vi "F Dwf Analog Out Node Frequency Info.vi"(6 "phzMax":dbl, 7 "phzMin":dbl, 8 "error in (no error)":errorcluster, 9 "node":i32, 10 "idxChannel":i32, 11 "hdwf":i32) -> (0 "error out":errorcluster, 3 "function return":i32, 4 "phzMax out":dbl, 5 "phzMin out":dbl)   [LabVIEW 2024, in "Olasdwf.lvlib"]
doc: "DWFAPI int FDwfAnalogOutNodeFrequencyInfo(HDWF hdwf, int idxChannel, AnalogOutNode node, double *phzMin, double *phzMax);"
uses:
  Olasdwf.lvlib
  Windows/System32/dwf.dll
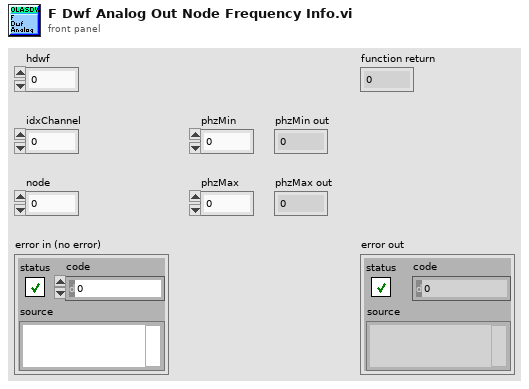
[diagram p1: front panel]
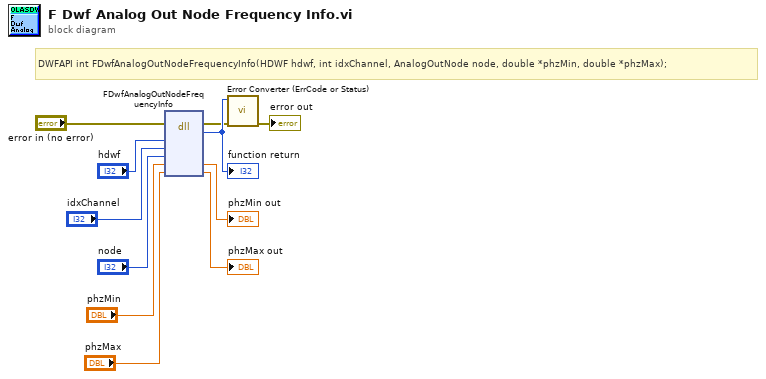
[diagram p0: block diagram]
diagram:
  # "DWFAPI int FDwfAnalogOutNodeFrequencyInfo(HDWF hdwf, int idxChannel, AnalogOutNode node, double *phzMin, double *phzMax);"
  n1 = dll-call lib="/Windows/System32/dwf.*" fn="FDwfAnalogOutNodeFrequencyInfo"(error in="error in (no error)", "hdwf"="hdwf", "idxChannel"="idxChannel", "node"="node", "phzMin"="phzMin", "phzMax"="phzMax") -> (error out=w2:errorcluster, w11:i32, "phzMin"=→"phzMin out":dbl, "phzMax"=→"phzMax out":dbl)  [unwired: 5 in, 1 out]
  "function return" <- w11
  n2 = call "Error Converter (ErrCode or Status).vi"("error in (no error)"=w2, "error code"=w11) -> ("error out"=→"error out":errorcluster)  [unwired: 9 in]
